vi "Quantizer (DBL Array).vi"(2 "quantization interval":dbl=0.1 format="%.2f", 3 "Input Points":dbl[](array[numeric]) format="%.2f") -> (1 "Output Points":dbl[](array[numeric]) format="%.2f")   [LabVIEW 2020, in "NI_AdvCtrl_nonlinear.lvlib"]
doc: "LabVIEW no longer supports this VI. You can obtain similar functionality by installing the LabVIEW Simulation Module.\n\nQuantizes an input signal. It is output=[input/quantization interval]*quantization interval."
uses:
  <vilib>/addons/control/advanced/NI_AdvCtrl_nonlinear.lvlib
  <vilib>/addons/control/advanced/NI_AdvCtrl_continuous linear.lvlib
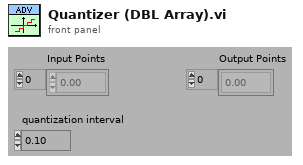
[diagram p1: front panel]
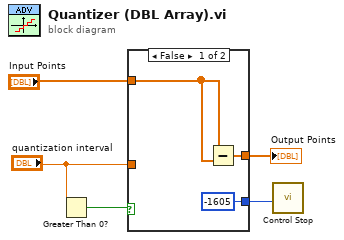
[diagram p0: block diagram]
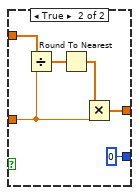
[diagram p2: hidden frame]
diagram:
  n1 = Greater Than 0?(x="quantization interval") -> (x > 0?=w4:bool)
  n2 = case shown="False" w4 {
    tunnel: [w6 w14] -> w2
    tunnel: "Input Points" -> [w7 w11]
    tunnel: "quantization interval" -> [_ w10]
    tunnel: [-1605 ("error") 0 ("error")] -> w1
    frame False {
      n3 = Subtract(x=w7, y=w7) -> (x-y=w6:dbl[])
    }
    frame True {
      n4 = Divide(x=w11, y=w10) -> (x/y=w12:dbl[])
      n5 = Round To Nearest(number=w12) -> (nearest integer value=w13:dbl[])
      n6 = Multiply(x=w13, y=w10) -> (x*y=w14:dbl[])
    }
  }
  "Output Points" <- w2
  n7 = call <vilib>:"Control Stop.vi"("error"=w1) -> ()  [unwired: 2 out]
